vi "Avoid Obstacle.vi"(9 "Robot Frame (World)":cluster{"X":sgl, "Y":sgl, "Theta":dbl}, 10 "Posture In":dbl[](array[numeric]), 11 "IF readings\n(meters)":dbl[](array[numeric]) format="%_6g") -> (3 "Frame Velocity":dbl[](array[numeric]))   [LabVIEW 2016]
uses:
  <vilib>/Analysis/coordinate.llb/Angle Range (Degree).ctl
  <vilib>/Analysis/coordinate.llb/Angle Units.ctl
  <vilib>/Analysis/coordinate.llb/Wrap Angle (scalar).vi
  <vilib>/addons/control/pid/pid.llb/PID (DBL).vi
  <vilib>/Analysis/NI_AAL_Angle.lvlib
  <vilib>/addons/control/pid/NI_PID_pid.lvlib
panel:
  out "atan2(y,x)":dbl
  out "x-y":dbl
  in  "V forward":dbl
  out "output":dbl format="%.2f"
  in  "PID gains":T1={"proportional gain (Kc)"=1.0, "integral time (Ti, min)"=0.01, "derivative time (Td, min)"=0.0} {"derivative time (Td, min)" format="%.3f"; "integral time (Ti, min)" format="%.3f"; "proportional gain (Kc)" format="%.3f"}
  in  "Sensor Gain":dbl[](array[numeric])=[1.0, 1.0, 0.5, 1.0, 1.0]
  out "ir distances wf":dbl[][](array[numeric])
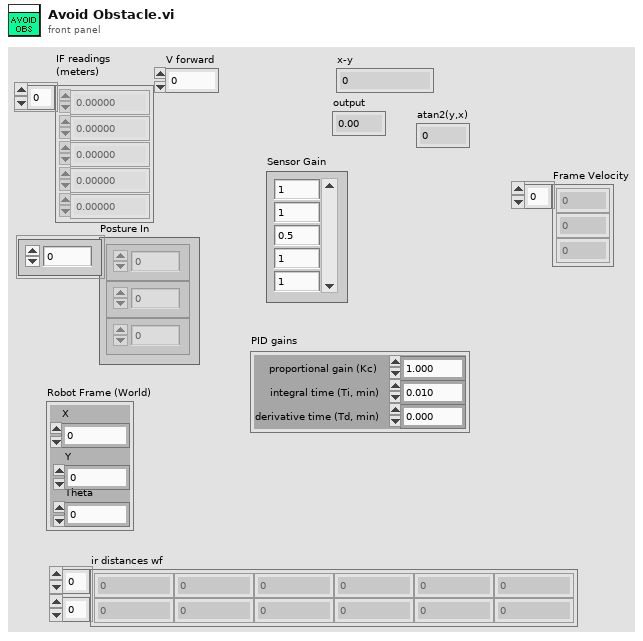
[diagram p1: front panel]
types:
  T1 = cluster{"proportional gain (Kc)":dbl, "integral time (Ti, min)":dbl, "derivative time (Td, min)":dbl}
  T2 = typedef "NI_AAL_Angle.lvlib/Angle Units.ctl" = i32
  T3 = typedef "NI_AAL_Angle.lvlib/Angle Range (Degree).ctl" = u16
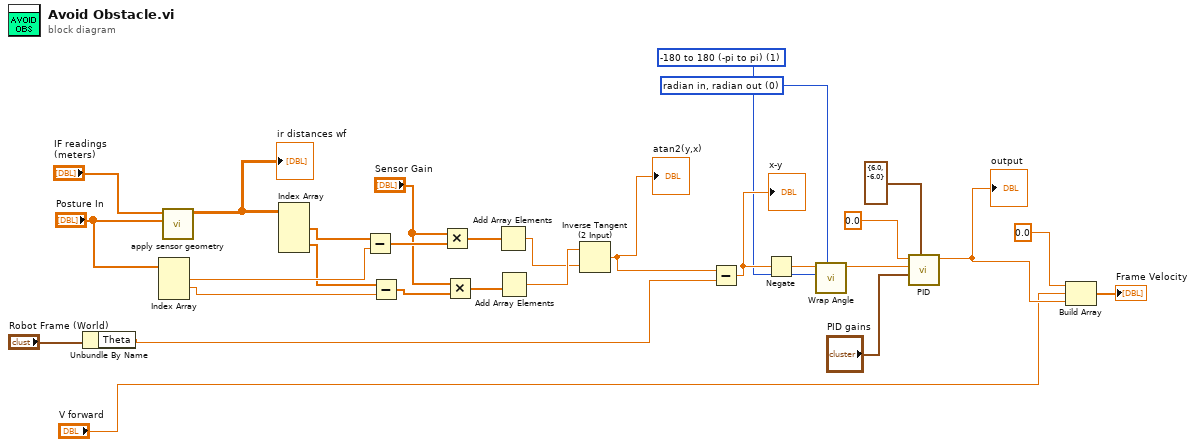
[diagram p0: block diagram]
diagram:
  w12 = T2 0 items=["radian in, radian out", "radian in, degree out", "degree in, degree out", "degree in, radian out"] ("angle units")
  w13 = T3 1 items=["none", "-180 to 180 (-pi to pi)", "0 to 360 (0 to 2pi)"] ("angle range")
  n1 = Unbundle By Name("Robot Frame (World)") -> ("Theta"=w2:dbl)
  n2 = Index Array(array="Posture In") -> (element #1=w25:dbl, element #2=w23:dbl)  [unwired: 3 in, 1 out]
  n3 = call "apply sensor geometry.vi"("Posture In"="Posture In", "IF readings\n(meters)"="IF readings\n(meters)") -> ("ir distances wf"=w27:dbl[][])  [unwired: 8 in, 1 out]
  "ir distances wf" <- w27
  n4 = Index Array(array=w27) -> (element #1=w26:dbl[], element #2=w24:dbl[])  [unwired: 4 in]
  n5 = Subtract(x=w26, y=w25) -> (x-y=w22:dbl[])
  n6 = Subtract(x=w24, y=w23) -> (x-y=w21:dbl[])
  n7 = Multiply(x="Sensor Gain", y=w22) -> (x*y=w19:dbl[])
  n8 = Multiply(x="Sensor Gain", y=w21) -> (x*y=w18:dbl[])
  n9 = Add Array Elements(numeric array=w19) -> (sum=w16:dbl)
  n10 = Add Array Elements(numeric array=w18) -> (sum=w17:dbl)
  n11 = Inverse Tangent (2 Input)(1:w16, 2:w17) -> (0:w15:dbl)
  "atan2(y,x)" <- w15
  n12 = Subtract(x=w15, y=w2) -> (x-y=w14:dbl)
  "x-y" <- w14
  n13 = Negate(x=w14) -> (-x=w1:dbl)
  n14 = call-poly <vilib>:"Wrap Angle.vi"("angle units"=w12, "angle range"=w13, "angle in"=w1) -> ("angle out"=w11:dbl)  [unwired: 7 in, 1 out]
  n15 = call-poly <vilib>:"PID.vi"("output range"=cluster{"output high":dbl, "output low":dbl} {"output high"=6.0, "output low"=-6.0}, "PID gains"="PID gains", "process variable"=w11, "setpoint"=0.0) -> ("output"=w7:dbl)  [unwired: 6 in, 1 out]
  "output" <- w7
  n16 = Build Array(0.0 ("element"), "V forward", w7) -> (→"Frame Velocity":dbl[])
